vi "sine run test.vi"() -> ()   [LabVIEW 2015]
uses:
  <vilib>/Platform/TimedLoop/XDataNode/timing_clust.ctl
  <vilib>/Platform/TimedLoop/XDataNode/nitl_modes.ctl
  <vilib>/Platform/TimedLoop/XDataNode/wakeup.ctl
  <vilib>/platform/TimedLoop/XDataNode/XDataNode.xnode
  <vilib>/Platform/TimedLoop/XDataNode/XDNodeRunTimeDep.lvlib
panel:
  out "x-y":dbl
  out "Waveform Chart":dbl(graph)
  out "current time":timestamp
  in  "Stop Button":bool
  out "x+y":dbl
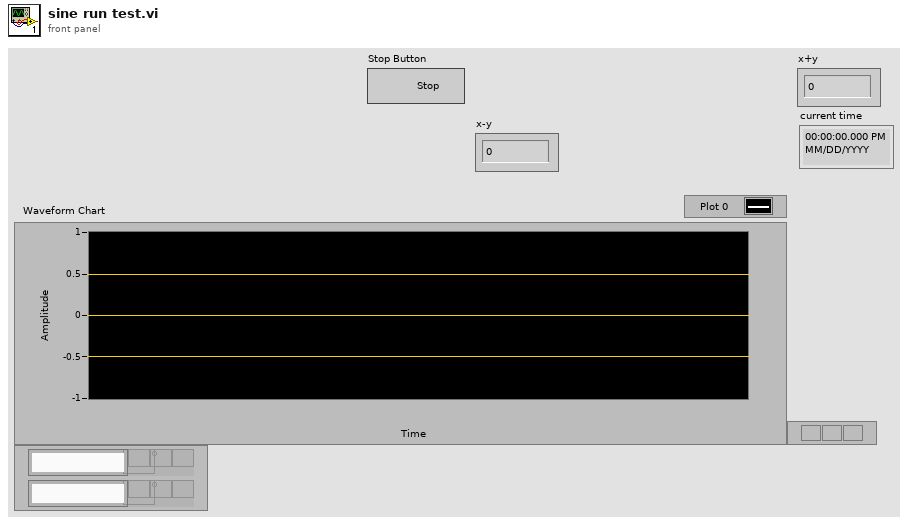
[diagram p1: front panel]
types:
  T1 = typedef "XDNodeRunTimeDep.lvlib/timing_clust.ctl" = cluster{"Expected End [f-1]":u64, "Actual End [f-1]":u64, "Finished Late? [f-1]":bool, "Expected End [i-1]":u64, "Actual End [i-1]":u64, "Finished Late? [i-1]":bool, "Expected Start [i]":u64, "Actual Start [i]":u64, "Expected Start [f]":u64, "Actual Start [f]":u64, "Source Name":string, "Structure Name":string, "Period":i64, "Deadline":i64, "Offset":i64, "Start":i64, "Priority":i32, "Timeout":i32, "Mode":T2, "Wakeup Reason":T3, "Error":errorcluster, "Source Type":string, "Secondary Source Type":string, "Global End Time":u64, "Global Start Time":u64, "Frame Duration":u64, "Iteration Duration":u64, "Assigned CPU":i32, "I/O Scan Engine Mode":u32}
  T2 = typedef "XDNodeRunTimeDep.lvlib/nitl_modes.ctl" = enum32{"No Change", "Process missed periods, maintain original phase", "Discard missed periods, maintain original phase", "Process missed periods, ignore original phase", "Discard missed periods, ignore original phase"}
  T3 = typedef "XDNodeRunTimeDep.lvlib/wakeup.ctl" = enum32{"Normal", "Aborted", "Asynchronous wakeup", "Timing source error", "Timed loop error", "Timeout"}
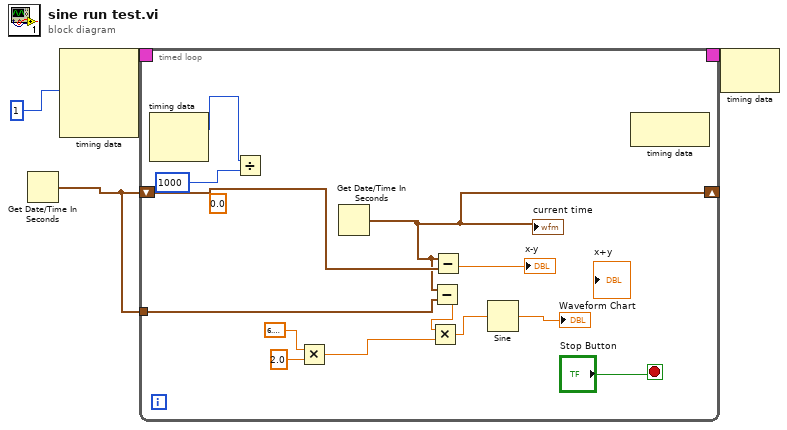
[diagram p0: block diagram]
diagram:
  n1 = Get Date/Time In Seconds() -> (seconds since 1Jan1904=w1:timestamp)
  n2 = node-c288(i64 1 ("Period")) -> (w4:T1)  [unwired: 3 in]
  n3 = timed-loop {
    timing: w4 -> [_]
    timing-out: [_] -> w3
    shift-right: [w10] -> _
    shift-left: w1 -> [w15]
    tunnel: w1 -> [w9]
    stop <- "Stop Button" stop-if-true
    (unwired) 0.0 ("phase")
    n4 = node-c288() -> (w17:i64)  [unwired: 1 in, 1 out]
    n5 = Divide(x=w17, y=i64 1000) -> ()  [unwired: 1 out]
    n6 = Multiply(x=6.283185307179586, y=2.0) -> (x*y=w7:dbl)
    n7 = Get Date/Time In Seconds() -> (seconds since 1Jan1904=w10:timestamp)
    "current time" <- w10
    n8 = Subtract(x=w10, y=w9) -> (x-y=w8:dbl)
    n9 = Multiply(x=w8, y=w7) -> (x*y=w6:dbl)
    n10 = Subtract(x=w10, y=w15) -> (x-y=→"x-y":dbl)
    n11 = Sine(x=w6) -> (sin(x)=→"Waveform Chart":dbl)
    n12 = node-c288() -> ()  [unwired: 1 in, 1 out]
  }
  n13 = node-c288(w3) -> ()  [unwired: 1 out]
